vi "_PC_D999_Get_Data.vi"(8 "error in (no error)":errorcluster) -> (0 "error IO":errorcluster, 1 "Value Array":dbl[](array[numeric]), 2 "Label array":string[](array[string]), 3 "Port array":string[](array[string]), 4 "timestamp":timestamp, 6 "index":u8)   [LabVIEW 2018]
uses:
  RT/PublicSubVI/Ctl/_ctl_RT_D999_Format.ctl
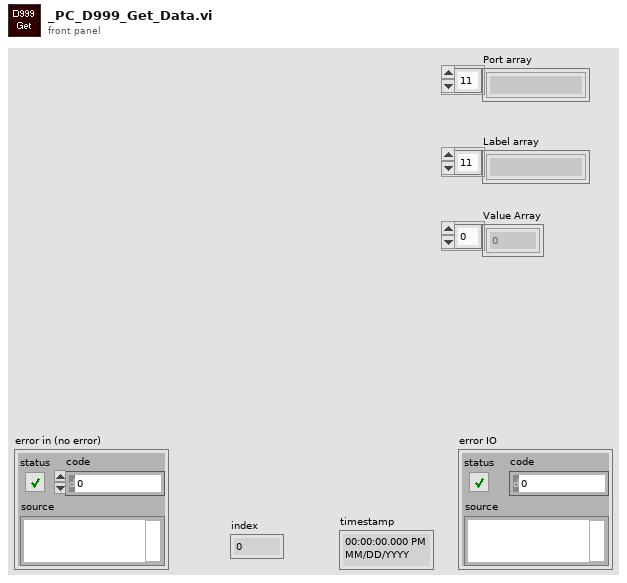
[diagram p1: front panel]
types:
  T1 = typedef "_ctl_RT_D999_Format.ctl" = cluster{"Port":string, "Label":string, "Value":dbl}[]
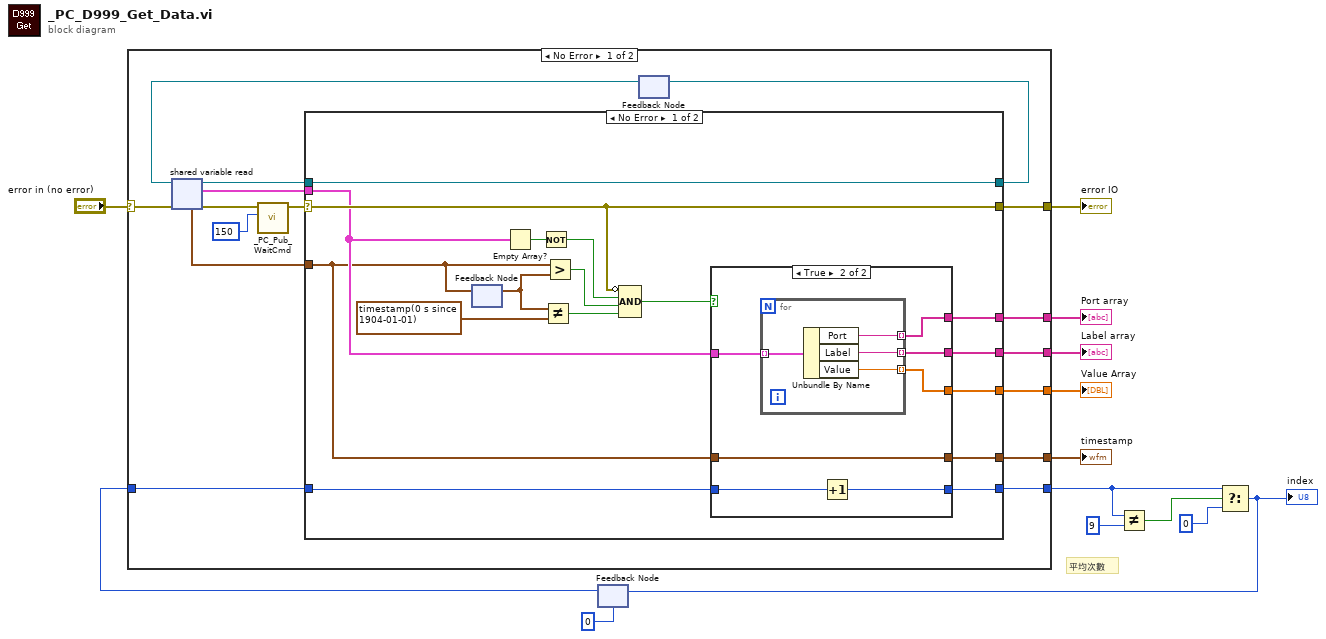
[diagram p0: block diagram]
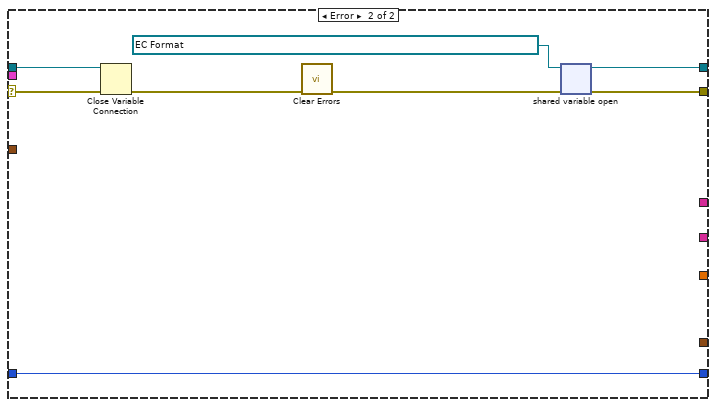
[diagram p3: hidden frame]
diagram:
  # "平均次數"
  n1 = feedback #1(u8 0) -> (w7:u8)
  n2 = case shown="No Error" "error in (no error)" {
    selector: "error in (no error)" -> [w29 w69]
    tunnel: [w24 _] -> w12
    tunnel: [w23 _] -> w11
    tunnel: [w22 _] -> w9
    tunnel: [w21 _] -> w10
    tunnel: [w20 w69] -> w8
    tunnel: [w15 w68] -> w3
    tunnel: w7 -> [w14 w68]
    frame No Error {
      n3 = feedback #2() -> (w25:refnum<k21>)  [unwired: 1 in]
      n4 = shared-variable-read(w25, w29) -> (w28:refnum<k21>, w18:errorcluster, w27:T1, w19:timestamp)
      n5 = call "_PC_Pub_WaitCmd.vi"("milliseconds to wait"=u32 150, "error in (no error)"=w18) -> ("error out"=w17:errorcluster)  [unwired: 9 in]
      n6 = case shown="No Error" w17 {
        selector: w17 -> [w41 w66]
        tunnel: w28 -> [w46 w67]
        tunnel: w27 -> [w39 _]
        tunnel: [w46 w62] -> w26
        tunnel: [w41 w61] -> w20
        tunnel: [w33 _] -> w24
        tunnel: [w38 _] -> w21
        tunnel: [w37 _] -> w22
        tunnel: [w36 _] -> w23
        tunnel: w19 -> [w32 _]
        tunnel: [w30 w60] -> w15
        tunnel: w14 -> [w31 w60]
        frame No Error {
          n7 = feedback #3() -> (w34:timestamp)  [unwired: 1 in]
          n8 = feedback-in #3(w32) -> ()
          n9 = Empty Array?(array=w39) -> (empty?=w45:bool)
          n10 = Not(x=w45) -> (.not. x?=w42:bool)
          n11 = Not Equal?(x=w34, y=timestamp(0 s since 1904-01-01)) -> (x != y?=w44:bool)
          n12 = Greater?(x=w32, y=w34) -> (0:w43:bool)
          n13 = Compound Arithmetic op=AND(invert w41, w42, w43, w44) -> (w40:bool)
          n14 = case shown="True" w40 {
            tunnel: [_ w54] -> w37
            tunnel: [_ w53] -> w36
            tunnel: w39 -> [_ w55]
            tunnel: [_ w52] -> w38
            tunnel: [w48 w51] -> w33
            tunnel: w32 -> [w48 w51]
            tunnel: w31 -> [w47 w50]
            tunnel: [w47 w49] -> w30
            frame False {
            }
            frame True {
              n15 = for {
                tunnel: w55 -> [w59] mode=indexing
                tunnel: [w58] -> w52 mode=indexing
                tunnel: [w57] -> w54 mode=indexing
                tunnel: [w56] -> w53 mode=indexing
                n16 = Unbundle By Name(w59) -> ("Port"=w58:string, "Label"=w57:string, "Value"=w56:dbl)
              }
              n17 = Increment(x=w50) -> (x+1=w49:u8)
            }
          }
        }
        frame Error {
          n18 = Close Variable Connection(8:w66, 11:w67) -> (0:w65:errorcluster)
          n19 = call <vilib>:"Clear Errors.vi"("error in (no error)"=w65) -> ("error out"=w64:errorcluster)  [unwired: 5 in, 1 out]
          n20 = shared-variable-open(refnum<k21> "ni.var.psp://NI-sbRIO/_RT_CtrlLoop_D999_Variables/D999_AI_Value" ("shared variable refnum in"), w64) -> (w62:refnum<k21>, w61:errorcluster)
        }
      }
      n21 = feedback-in #2(w26) -> ()
    }
    frame Error {
    }
  }
  "error IO" <- w8
  "Label array" <- w9
  "Value Array" <- w11
  "Port array" <- w10
  "timestamp" <- w12
  n22 = Not Equal?(x=w3, y=u8 9) -> (x != y?=w4:bool)
  n23 = Select(t=w3, s=w4, f=u8 0) -> (s? t:f=w2:u8)
  "index" <- w2
  n24 = feedback-in #1(w2) -> ()
